vi "currentExperimentSettings.vi"(5 "error in (no error)":errorcluster) -> (10 "Last Name":string, 12 "Last Description":string, 13 "Experiment settings ID":i64, 14 "output cluster 2":T1, 16 "Last Group ID":i32, 19 "error out":errorcluster)   [LabVIEW 2012]
doc: "Displays a standard dialog box that prompts users to enter information, such as a user name and password.\n--------------------\n\nThis Express VI is configured as follows:\n\nMessage to Display to the User:Please Enter Experiment Settings Information For Database Storage.\nThe inputs are: \nNumber: Please Enter Group ID\nText Entry Box: Please Enter Tags:\nText Entry Box: Please Enter Experiment Description:"
uses:
  Public API/DisplayExperimentSetting.ctl
  Public API/ExperimentSetting.ctl
  <vilib>/addons/database/Connection.llb/Conn Execute.vi
  <vilib>/addons/database/Recordset.llb/Rec Fetch Recordset Data (R).vi
  <vilib>/addons/database/Recordset.llb/Rec Destroy - Connection.vi
  <vilib>/addons/database/_DB Variant To Data/Database Variant To Data.xnode
  <vilib>/addons/database/NI_Database_API.lvlib
panel:
  # "Experiment Status:"
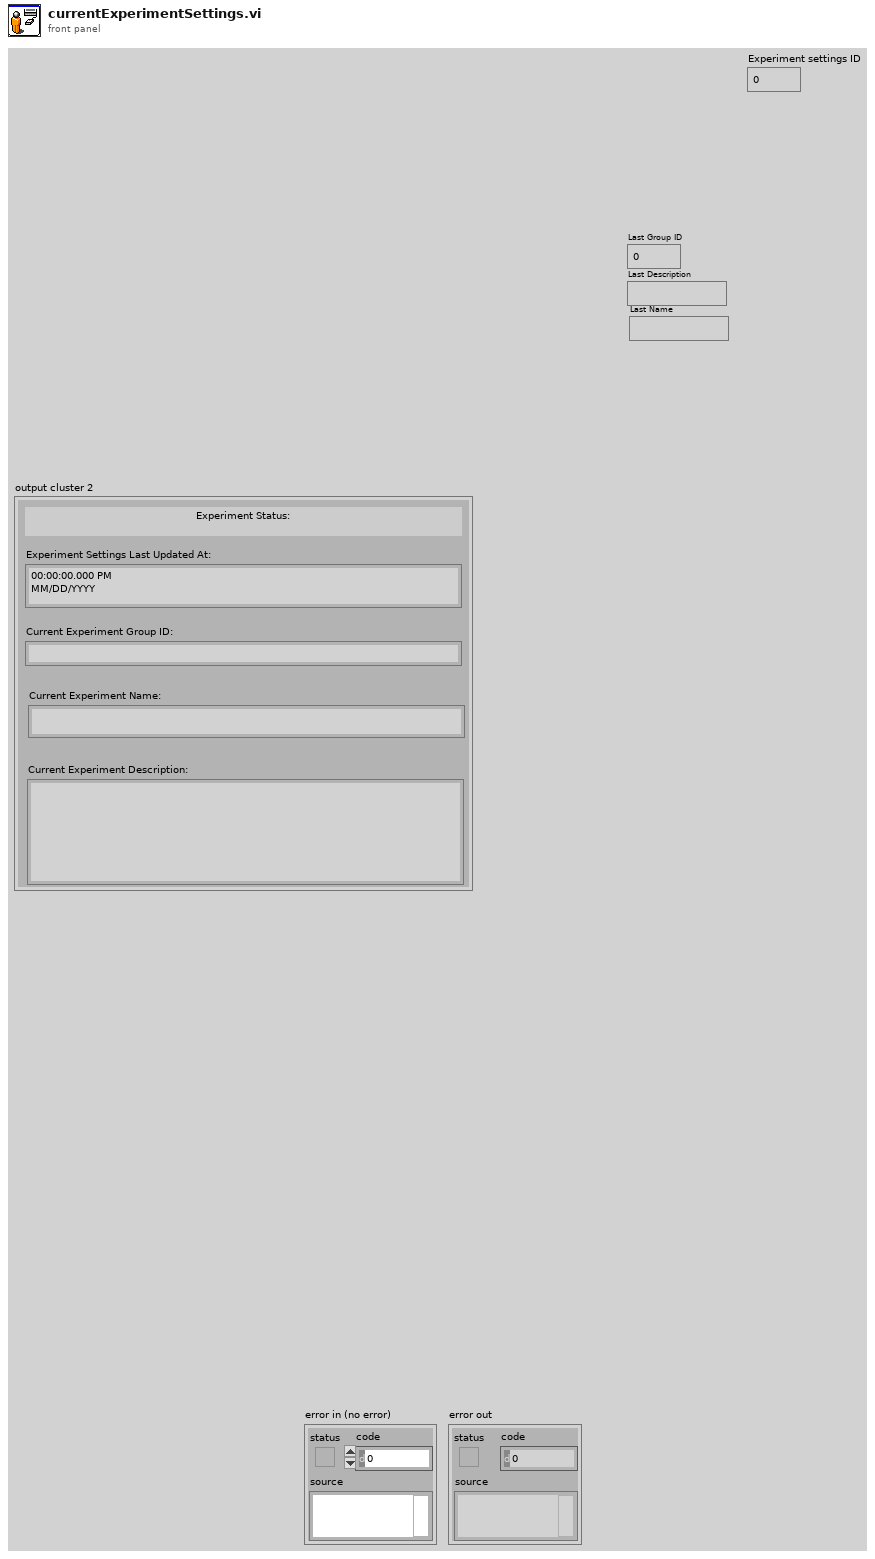
[diagram p1: front panel]
types:
  T1 = typedef "DisplayExperimentSetting.ctl" = cluster{"Current Experiment Name:":string, "Current Experiment Description:":string, "Current Experiment Group ID:":string, "Experiment Settings Last Updated At:":timestamp}
  T2 = cluster{"Input Name":string, "Input Data Type":i32}
  T3 = typedef "NI_Database_API.lvlib/Conn ObjectReference.ctl" = refnum<k1>
  T4 = typedef "NI_Database_API.lvlib/Rec ObjectReference.ctl" = refnum<k1>
  T5 = typedef "ExperimentSetting.ctl" = cluster{"Experiment Settings  ID":i64, "Time Stamp":i64, "Group ID":i32, "Tags:":string, "Description:":string}
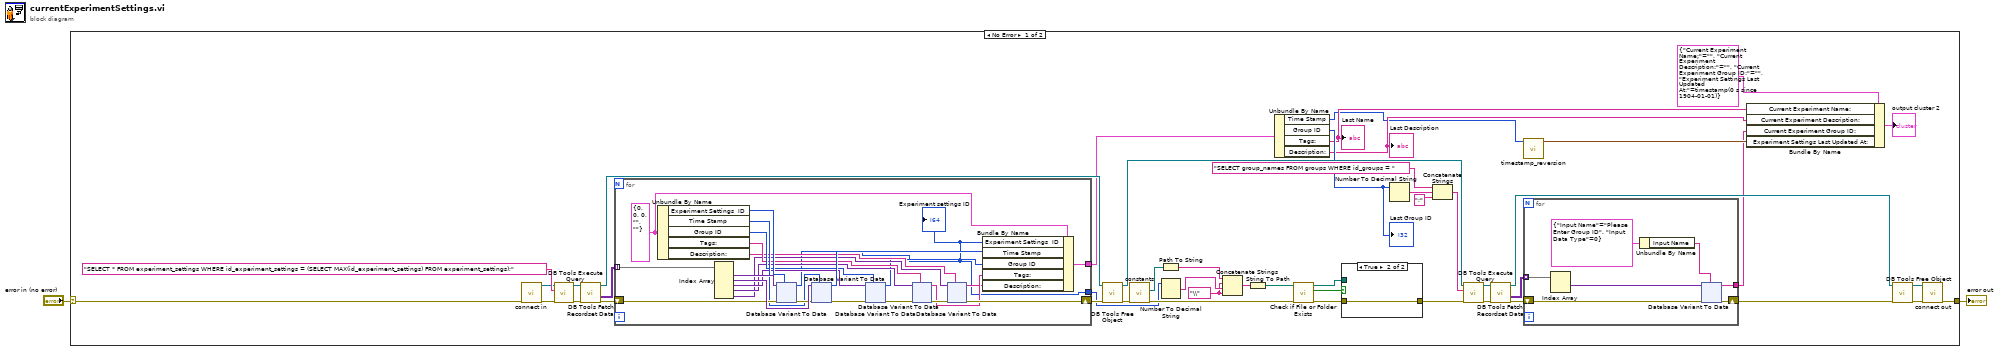
[diagram p0: block diagram]
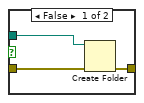
[diagram p2: hidden frame]
diagram:
  n1 = case shown="No Error" "error in (no error)" {
    selector: "error in (no error)" -> [w42 w276]
    tunnel: [w28 w276] -> w1
    frame No Error {
      w8 = "\\"
      n2 = call "connect in.vi"("error in (no error)"=w42) -> ("error out"=w43:errorcluster, "Database Connection"=w40:T3)  [unwired: 6 in, 1 out]
      n3 = call-poly <vilib>:"DB Tools Execute Query.vi"("error in (no error)"=w43, "SQL query"="SELECT * FROM experiment_settings WHERE id_experiment_settings = (SELECT MAX(id_experiment_settings) FROM experiment_settings);", "connection reference"=w40) -> ("error out"=w45:errorcluster, "recordset reference"=w44:T4)  [unwired: 5 in]
      n4 = call-poly <vilib>:"DB Tools Fetch Recordset Data.vi"("error in (no error)"=w45, "recordset reference"=w44) -> ("error out"=w48:errorcluster, "recordset data"=w47:variant[][], "recordset reference out"=w39:T4)  [unwired: 3 in]
      n5 = for {
        tunnel: w47 -> [w115] mode=indexing
        shift-right: [w102] -> w41
        shift-left: w48 -> [w111]
        tunnel: [w106] -> w38
        tunnel: [w92] -> w10
        w107 = T5 {"Experiment Settings  ID"=0, "Time Stamp"=0, "Group ID"=0, "Tags:"="", "Description:"=""} ("Experiment Settings")
        n6 = Unbundle By Name(w107) -> ("Experiment Settings  ID"=w110:i64, "Time Stamp"=w108:i64, "Group ID"=w101:i32, "Tags:"=w99:string, "Description:"=w97:string)
        n7 = Index Array(array=w115) -> (element #1=w114:variant, element #2=w113:variant, element #3=w100:variant, element #4=w98:variant, element #5=w96:variant)  [unwired: 5 in]
        n8 = xnode "Database Variant To Data"("database variant"=w114, "error in"=w111, "type"=w110) -> ("data"=w92:i64, "error out"=w112:errorcluster)
        "Experiment settings ID" <- w92
        n9 = xnode "Database Variant To Data"("database variant"=w113, "error in"=w112, "type"=w108) -> ("data"=w109:i64, "error out"=w105:errorcluster)
        n10 = xnode "Database Variant To Data"("database variant"=w100, "error in"=w105, "type"=w101) -> ("data"=w95:i32, "error out"=w104:errorcluster)
        n11 = xnode "Database Variant To Data"("database variant"=w98, "error in"=w104, "type"=w99) -> ("data"=w94:string, "error out"=w103:errorcluster)
        n12 = xnode "Database Variant To Data"("database variant"=w96, "error in"=w103, "type"=w97) -> ("data"=w93:string, "error out"=w102:errorcluster)
        n13 = Bundle By Name(cluster=w107, "Experiment Settings  ID"=w92, "Time Stamp"=w109, "Group ID"=w95, "Tags:"=w94, "Description:"=w93) -> (w106:T5)
      }
      n14 = call-poly <vilib>:"DB Tools Free Object.vi"("error in (no error)"=w41, "recordset reference"=w39) -> ("error out"=w9:errorcluster, "connection reference"=w31:T3)  [unwired: 8 in]
      n15 = call "constants.vi"("error in (no error)"=w9) -> ("error out"=w11:errorcluster, "file path for Signal .hdf5 files"=w6:path)  [unwired: 4 in, 5 out]
      n16 = Path To String(path=w6) -> (string=w5:string)
      n17 = Number To Decimal String(number=w10) -> (decimal integer string=w15:string)  [unwired: 1 in]
      n18 = Concatenate Strings(w5, w8, w15, w8) -> (w4:string)
      n19 = String To Path(string=w4) -> (path=w3:path)
      n20 = Unbundle By Name(w38) -> ("Time Stamp"=w19:i64, "Group ID"=w24:i32, "Tags:"=w21:string, "Description:"=w20:string)
      "Last Group ID" <- w24
      "Last Description" <- w20
      "Last Name" <- w21
      n21 = call <vilib>:"Check if File or Folder Exists.vi"("error in (no error)"=w11, "path"=w3) -> ("error out"=w12:errorcluster, "file or folder exists?"=w14:bool, "dup path"=w13:path)  [unwired: 7 in]
      n22 = case shown="True" w14 {
        tunnel: w13 -> [w51 _]
        tunnel: w12 -> [w50 w52]
        tunnel: [w49 w52] -> w7
        frame False {
          n23 = Create Folder(path (use dialog)=w51, error in=w50) -> (error out=w49:errorcluster)  [unwired: 1 in, 2 out]
        }
        frame True {
        }
      }
      n24 = Number To Decimal String(number=w24) -> (decimal integer string=w26:string)  [unwired: 1 in]
      n25 = Concatenate Strings("SELECT group_names FROM groups WHERE id_groups = " ("SQL query"), w26, ";" ("string")) -> (w23:string)
      n26 = call-poly <vilib>:"DB Tools Execute Query.vi"("error in (no error)"=w7, "SQL query"=w23, "connection reference"=w31) -> ("error out"=w35:errorcluster, "recordset reference"=w34:T4)  [unwired: 5 in]
      n27 = call-poly <vilib>:"DB Tools Fetch Recordset Data.vi"("error in (no error)"=w35, "recordset reference"=w34) -> ("error out"=w37:errorcluster, "recordset data"=w36:variant[][], "recordset reference out"=w30:T4)  [unwired: 3 in]
      n28 = call "timestamp_reversion.vi"("Integer Timestamp"=w19) -> ("time stamp"=w18:timestamp)  [unwired: 8 in, 1 out]
      n29 = for {
        tunnel: w36 -> [w57] mode=indexing
        shift-right: [w53] -> w29
        shift-left: w37 -> [w56]
        tunnel: [w54] -> w17
        n30 = Index Array(array=w57) -> (element #1=w59:variant)  [unwired: 2 in, 1 out]
        n31 = Unbundle By Name(T2 {"Input Name"="Please Enter Group ID", "Input Data Type"=0}) -> ("Input Name"=w58:string)
        n32 = xnode "Database Variant To Data"("database variant"=w59, "error in"=w56, "type"=w58) -> ("data"=w54:string, "error out"=w53:errorcluster)
      }
      n33 = Bundle By Name(cluster=T1 {"Current Experiment Name:"="", "Current Experiment Description:"="", "Current Experiment Group ID:"="", "Experiment Settings Last Updated At:"=timestamp(0 s since 1904-01-01)} ("Experiment Settings"), "Current Experiment Name:"=w21, "Current Experiment Description:"=w20, "Current Experiment Group ID:"=w17, "Experiment Settings Last Updated At:"=w18) -> (→"output cluster 2":T1)
      n34 = call-poly <vilib>:"DB Tools Free Object.vi"("error in (no error)"=w29, "recordset reference"=w30) -> ("error out"=w32:errorcluster, "connection reference"=w33:T3)  [unwired: 8 in]
      n35 = call "connect out.vi"("error in (no error)"=w32, "connection reference"=w33) -> ("error out"=w28:errorcluster)  [unwired: 9 in]
    }
    frame Error {
    }
  }
  "error out" <- w1
